vi "Calc Ip Iu dP.vi"(7 "init":bool, 8 "P start [MPa]":dbl, 9 "P end [MPa]":dbl, 10 "U":dbl, 11 "P":dbl) -> (0 "done":bool, 1 "delta P":dbl, 2 "integral U(t)":dbl format="%0.2f", 3 "integral P(t)":dbl format="%0.2f")   [LabVIEW 2019]
uses:
  <vilib>/ptbypt/NI_PtbyPt.lvlib
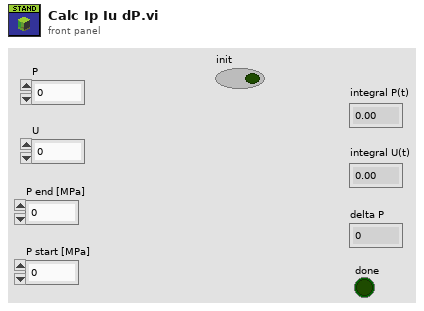
[diagram p1: front panel]
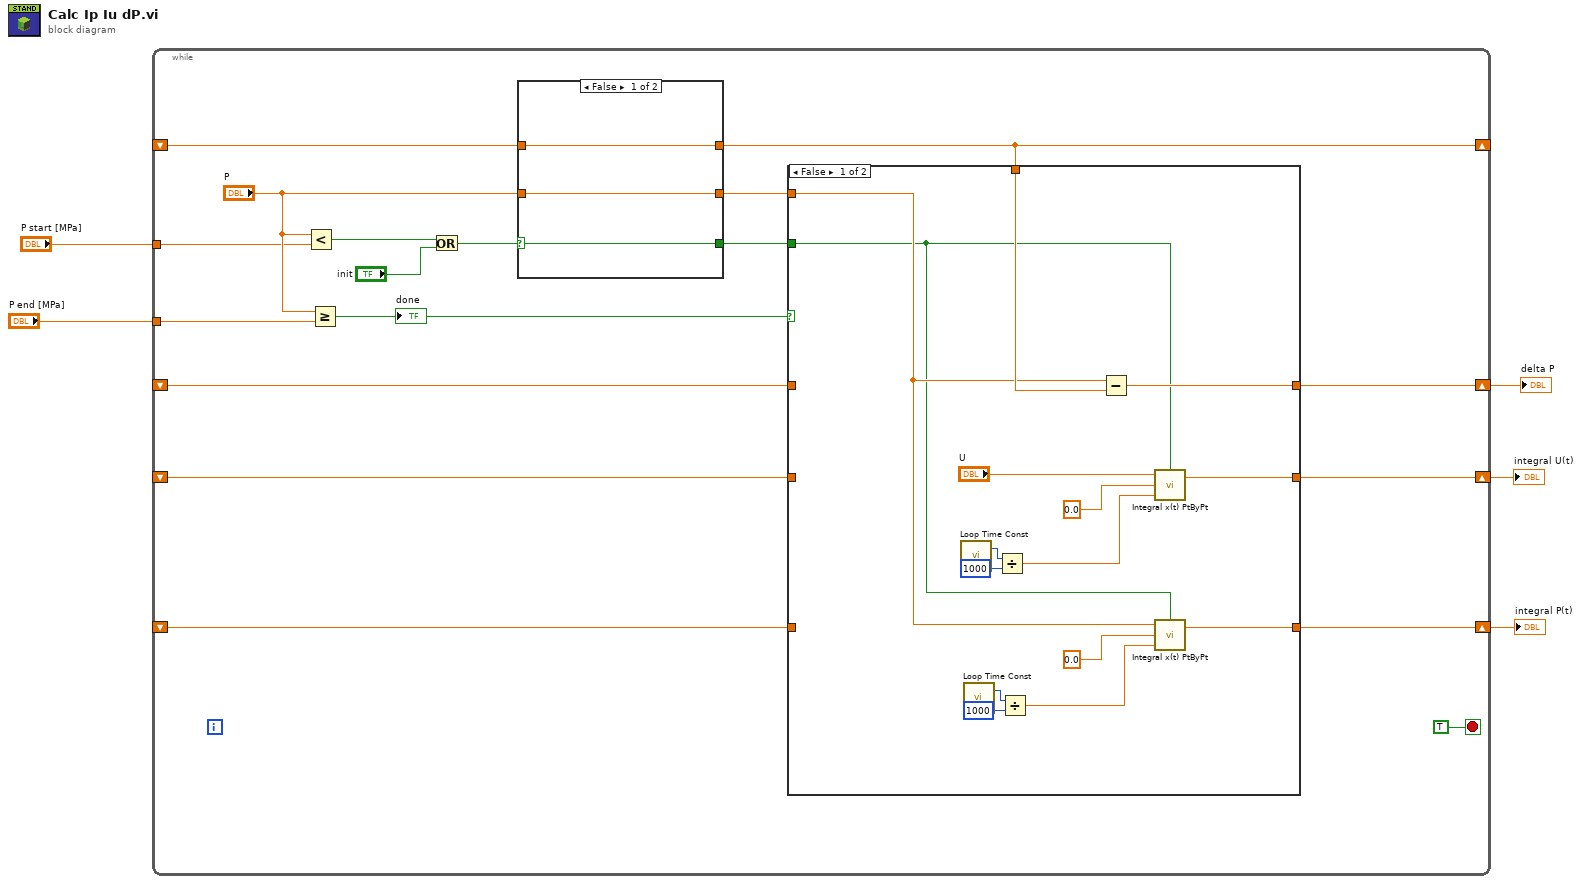
[diagram p0: block diagram]
diagram:
  n1 = while {
    shift-right: [w9] -> _
    shift-left: _ -> [w20]
    tunnel: "P start [MPa]" -> [w17]
    tunnel: "P end [MPa]" -> [w16]
    shift-right: [w15] -> w3
    shift-left: _ -> [w11]
    shift-right: [w14] -> w2
    shift-left: _ -> [w10]
    shift-right: [w8] -> w1
    shift-left: _ -> [w7]
    stop <- TRUE stop-if-true
    n2 = Less?(x="P", y=w17) -> (x < y?=w22:bool)
    n3 = Greater Or Equal?(x="P", y=w16) -> (x >= y?=w13:bool)
    "done" <- w13
    n4 = Or(x=w22, y="init") -> (x .or. y?=w19:bool)
    n5 = case shown="False" w19 {
      selector: w19 -> [w42 w45]
      tunnel: "P" -> [w44 w46]
      tunnel: [w44 w46] -> w12
      tunnel: [w43 w46] -> w9
      tunnel: w20 -> [w43 _]
      tunnel: [w42 w45] -> w6
      frame False {
      }
      frame True {
      }
    }
    n6 = case shown="False" w13 {
      tunnel: [w29 w41] -> w15
      tunnel: [w28 w40] -> w14
      tunnel: w12 -> [w26 _]
      tunnel: w11 -> [_ w41]
      tunnel: w10 -> [_ w40]
      tunnel: w9 -> [w27 _]
      tunnel: [w25 w39] -> w8
      tunnel: w7 -> [_ w39]
      tunnel: w6 -> [w24 _]
      frame False {
        n7 = call "Loop Time Const.vi"() -> ("loop time ms"=w38:i64)  [unwired: 3 in]
        n8 = call "Loop Time Const.vi"() -> ("loop time ms"=w31:i64)  [unwired: 3 in]
        n9 = Divide(x=w38, y=i64 1000) -> (x/y=w37:dbl)
        n10 = Divide(x=w31, y=i64 1000) -> (x/y=w30:dbl)
        n11 = Subtract(x=w26, y=w27) -> (x-y=w25:dbl)
        n12 = call <vilib>:"Integral x(t) PtByPt.vi"("initialize"=w24, "dt"=w37, "initial condition"=0.0, "x"="U") -> ("integral x(t)"=w29:dbl)  [unwired: 1 out]
        n13 = call <vilib>:"Integral x(t) PtByPt.vi"("initialize"=w24, "dt"=w30, "initial condition"=0.0, "x"=w26) -> ("integral x(t)"=w28:dbl)  [unwired: 1 out]
      }
      frame True {
      }
    }
  }
  "integral U(t)" <- w3
  "integral P(t)" <- w2
  "delta P" <- w1
